vi "Global stop DAQ.vi"() -> ()   [LabVIEW 2020]
panel:
  in  "Global stop DAQ":bool
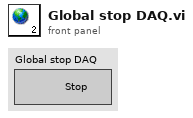
[diagram p1: front panel]
diagram:
